vi "Save Display Files.vi"(0 "Name":string, 5 "Spreadsheet String":string, 7 "base path":path, 9 "Display Array":string[][](array[string]), 11 "error in (no error)":errorcluster) -> (15 "error out":errorcluster)   [LabVIEW 2020]
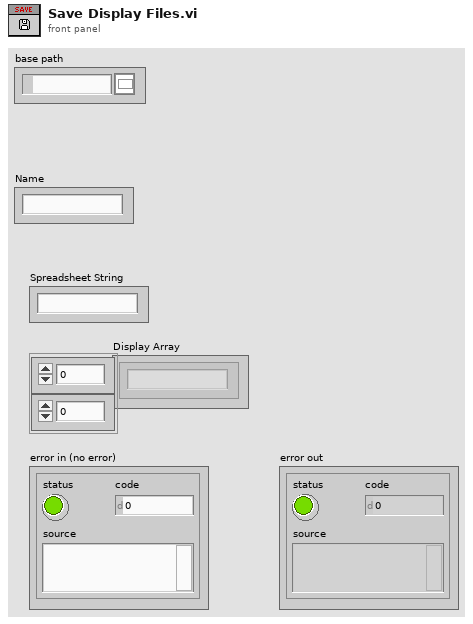
[diagram p1: front panel]
types:
  T1 = enum16{"open", "replace", "create", "open or create", "replace or create", "replace or create with confirmation"}
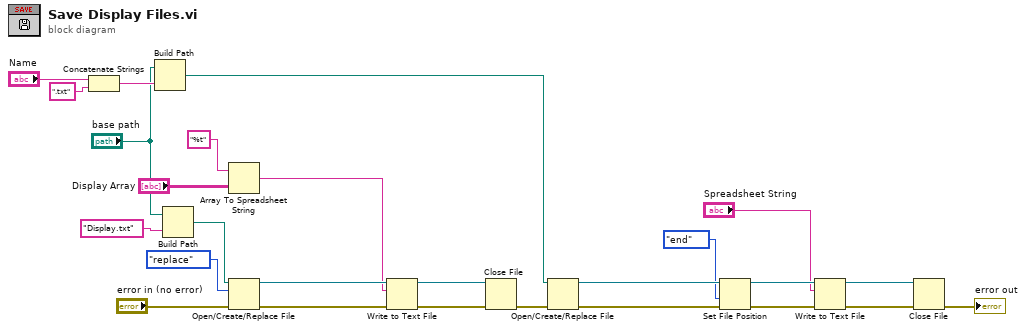
[diagram p0: block diagram]
diagram:
  n1 = Concatenate Strings("Name", ".txt" ("string")) -> (w5:string)
  n2 = Build Path(base path="base path", name or relative path=w5) -> (appended path=w7:path)
  n3 = Build Path(base path="base path", name or relative path="Display.txt") -> (appended path=w2:path)
  n4 = Array To Spreadsheet String(array="Display Array", 3:"%t" ("format string")) -> (spreadsheet string=w12:string)  [unwired: 1 in]
  n5 = Open/Create/Replace File(file path (use dialog)=w2, error in="error in (no error)", operation (0:open)=T1."replace") -> (refnum out=w18:refnum<file>, error out=w15:errorcluster)  [unwired: 3 in, 1 out]
  n6 = Write to Text File(file (use dialog)=w18, text=w12, error in=w15) -> (refnum out=w17:refnum<file>, error out=w16:errorcluster)  [unwired: 1 in, 1 out]
  n7 = Close File(refnum=w17, error in=w16) -> (error out=w21:errorcluster)  [unwired: 1 out]
  n8 = Open/Create/Replace File(file path (use dialog)=w7, error in=w21) -> (refnum out=w20:refnum<file>, error out=w22:errorcluster)  [unwired: 4 in, 1 out]
  n9 = Set File Position(refnum=w20, from (0:start)=enum16{"start", "end", "current"}."end", error in=w22) -> (refnum out=w11:refnum<file>, error out=w10:errorcluster)  [unwired: 1 in]
  n10 = Write to Text File(file (use dialog)=w11, text="Spreadsheet String", error in=w10) -> (refnum out=w24:refnum<file>, error out=w23:errorcluster)  [unwired: 1 in, 1 out]
  n11 = Close File(refnum=w24, error in=w23) -> (error out=→"error out":errorcluster)  [unwired: 1 out]
